vi "FlushPort.vi"(0 "reference":refnum<class "VdRs232.lvclass">, 5 "error in (no error)":errorcluster) -> (14 "duplicate reference":refnum<class "VdRs232.lvclass">, 16 "stringRead":string, 19 "error out":errorcluster)   [LabVIEW 2020, in "VdRs232.lvclass"]
doc: "Reads data from the com-port"
uses:
  VdRs232.lvclass
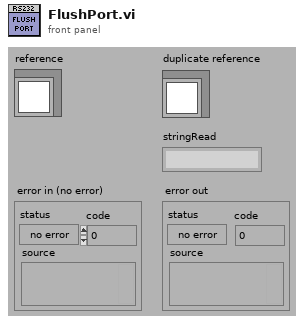
[diagram p1: front panel]
types:
  T1 = typedef "VdRs232.lvclass/ObjectAttributes.ctl" = cluster{"visaRef":refnum<visa-resource-name>, "portSetting":T2, "TimeoutTime(ms)":u32, "TerminationCharUsed":bool, "MatchPatternToIndicateCompleteResponse":string, "Creators":i32, "EndCharToSendForEveryMessage":string, "DefaultReadDataSize":u32, "SynchronousMode":bool, "Lock":T7}
  T2 = typedef "VdRs232.lvclass/ComParamsType.ctl" = cluster{"portNbr":T3, "baudRate":T4, "flowControl":T5, "parity":T6, "dataBits":u16, "stop bits (10: 1 bit)":u16}
  T3 = typedef "VdRs232.lvclass/VdRs232I_ComPortType.ctl" = enum16{"Com1", "Com2", "Com3", "Com4", "Com5", "Com6", "Com7", "Com8", "Com9", "Com10", "Com11", "Com12", "Com13", "Com14", "Com15", "Com16", "Com17", "Com18", "Com19", "Com20", "Com21", "Com22", "Com23", "Com24", "Com25", "Com26", "Com27", "Com28", "Com29", "Com30", "Com31", "Com32", "Com33", "Com34", "Com35", "Com36", "Com37", "Com38", "Com39", "Com40", "Com41", "Com42", "Com43", "Com44", "Com45", "Com46", "Com47", "Com48", "Com49", "Com50", "Com51", "Com52", "Com53", "Com54", "Com55", "Com56", "Com57", "Com58", "Com59", "Com60", "Com61", "Com62", "Com63", "Com64", "Com65", "Com66", "Com67", "Com68", "Com69", "Com70", "Com71", "Com72", "Com73", "Com74", "Com75", "Com76", "Com77", "Com78", "Com79", "Com80", "Com81", "Com82", "Com83", "Com84", "Com85", "Com86", "Com87", "Com88", "Com89", "Com90", "Com91", "Com92", "Com93", "Com94", "Com95", "Com96", "Com97", "Com98", "Com99", "Com100", "Com101", "Com102", "Com103", "Com104", "Com105", "Com106", "Com107", "Com108", "Com109", "Com110", "Com111", "Com112", "Com113", "Com114", "Com115", "Com116", "Com117", "Com118", "Com119", "Com120", "Com121", "Com122", "Com123", "Com124", "Com125", "Com126", "Com127", "Com128", "Com129", "Com130", "Com131", "Com132", "Com133", "Com134", "Com135", "Com136", "Com137", "Com138", "Com139", "Com140", "Com141", "Com142", "Com143", "Com144", "Com145", "Com146", "Com147", "Com148", "Com149", "Com150", "Com151", "Com152", "Com153", "Com154", "Com155", "Com156", "Com157", "Com158", "Com159", "Com160", "Com161", "Com162", "Com163", "Com164", "Com165", "Com166", "Com167", "Com168", "Com169", "Com170", "Com171", "Com172", "Com173", "Com174", "Com175", "Com176", "Com177", "Com178", "Com179", "Com180", "Com181", "Com182", "Com183", "Com184", "Com185", "Com186", "Com187", "Com188", "Com189", "Com190", "Com191", "Com192", "Com193", "Com194", "Com195", "Com196", "Com197", "Com198", "Com199", "Com200", "Com201", "Com202", "Com203", "Com204", "Com205", "Com206", "Com207", "Com208", "Com209", "Com210", "Com211", "Com212", "Com213", "Com214", "Com215", "Com216", "Com217", "Com218", "Com219", "Com220", "Com221", "Com222", "Com223", "Com224", "Com225", "Com226", "Com227", "Com228", "Com229", "Com230", "Com231", "Com232", "Com233", "Com234", "Com235", "Com236", "Com237", "Com238", "Com239", "Com240", "Com241", "Com242", "Com243", "Com244", "Com245", "Com246", "Com247", "Com248", "Com249", "Com250", "Com251", "Com252", "Com253", "Com254", "Com255"}
  T4 = typedef "VdRs232.lvclass/VdBaudRateType.ctl" = enum16{"1200", "2400", "9600", "14400", "19200", "28800", "38400", "57600", "115200", "230400", "460800", "691200", "921600"}
  T5 = typedef "VdRs232.lvclass/VdFlowControlType.ctl" = enum16{"None", "CTS/RTS", "XOn/XOff"}
  T6 = typedef "VdRs232.lvclass/VdParityType.ctl" = enum16{"None", "Odd", "Even"}
  T7 = typedef "Semaphore RefNum" = refnum<k1>
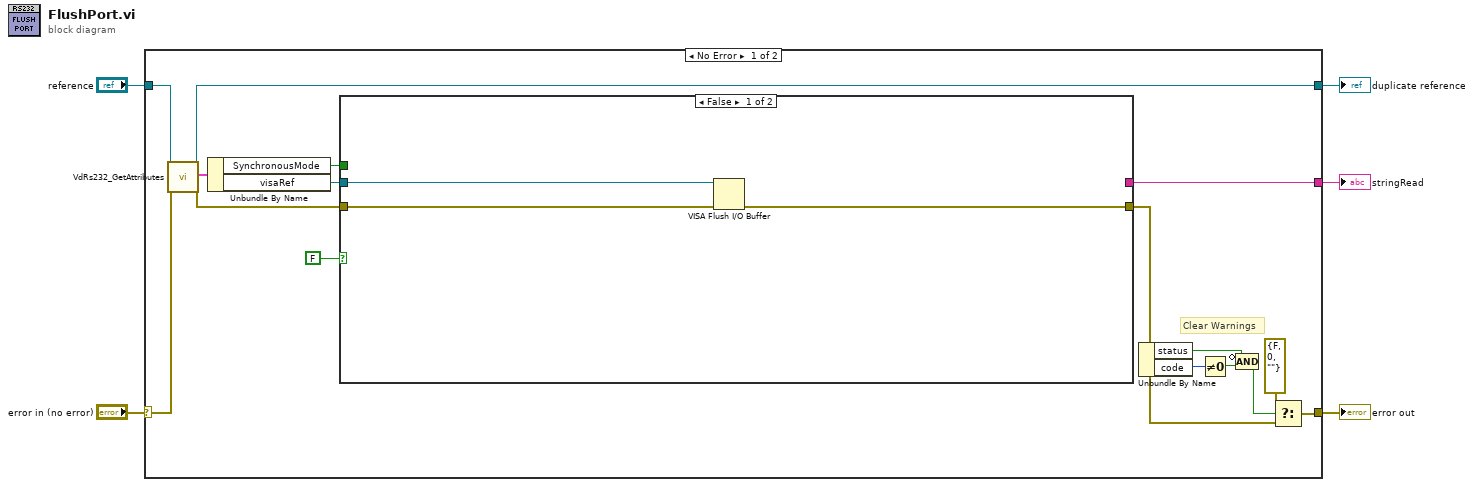
[diagram p0: block diagram]
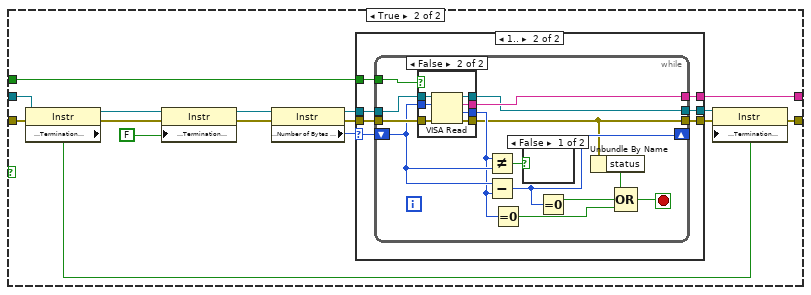
[diagram p2: hidden frame]
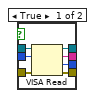
[diagram p4: hidden frame]
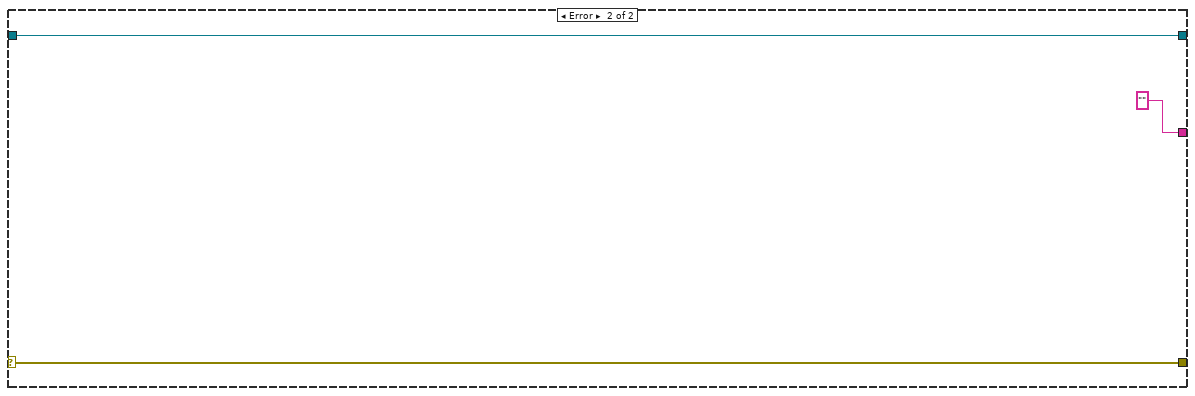
[diagram p6: hidden frame]
diagram:
  n1 = case shown="No Error" "error in (no error)" {
    selector: "error in (no error)" -> [w20 w79]
    tunnel: [w10 w79] -> w5
    tunnel: "reference" -> [w21 w80]
    tunnel: [w19 w80] -> w2
    tunnel: [w18 "" ("read buffer")] -> w1
    frame No Error {
      # "Clear Warnings"
      n2 = call "VdRs232_GetAttributes.vi"("reference in"=w21, "error in (no error)"=w20) -> ("reference out"=w19:refnum<class "VdRs232.lvclass">, "Data"=w6:T1, "error out"=w17:errorcluster)  [unwired: 1 in, 14 out]
      n3 = Unbundle By Name(w6) -> ("SynchronousMode"=w7:bool, "visaRef"=w16:refnum<visa-resource-name>)
      n4 = case shown="False" FALSE {
        tunnel: [_ w40] -> w18
        tunnel: w17 -> [w23 w39]
        tunnel: w16 -> [w24 w32]
        tunnel: [w22 w26] -> w11
        tunnel: w7 -> [_ w25]
        frame False {
          n5 = VISA Flush I/O Buffer(VISA resource name=w24, error in (no error)=w23) -> (error out=w22:errorcluster)  [unwired: 2 out]
        }
        frame True {
          n6 = property class="Instr"(reference=w32, error in=w39) -> (reference out=w30:refnum<visa-resource-name>, error out=w29:errorcluster, "Message Based Settings:Termination Character Enable"=w33:bool)
          n7 = property class="Instr"(reference=w30, error in=w29, "Message Based Settings:Termination Character Enable"=FALSE) -> (reference out=w28:refnum<visa-resource-name>, error out=w27:errorcluster)
          n8 = property class="Instr"(reference=w28, error in=w27) -> (reference out=w36:refnum<visa-resource-name>, error out=w37:errorcluster, "Serial Settings:Number of Bytes at Serial Port"=w38:u32)
          n9 = case shown="1.." w38 {
            selector: w38 -> [_ w44]
            tunnel: w36 -> [w41 w49]
            tunnel: w37 -> [w42 w48]
            tunnel: [_ w47] -> w40
            tunnel: [w42 w46] -> w34
            tunnel: [w41 w45] -> w35
            tunnel: w25 -> [_ w43]
            frame 0, Default {
            }
            frame 1.. {
              n10 = while {
                tunnel: w49 -> [w63]
                tunnel: w48 -> [w62]
                tunnel: [w61] -> w47
                tunnel: [w55] -> w46
                tunnel: [w60] -> w45
                shift-right: [w56] -> _
                shift-left: w44 -> [w58]
                tunnel: w43 -> [w50]
                stop <- w51 stop-if-true
                n11 = case shown="False" w50 {
                  tunnel: w63 -> [w70 w77]
                  tunnel: w62 -> [w69 w76]
                  tunnel: [w68 w75] -> w61
                  tunnel: [w67 w74] -> w60
                  tunnel: w58 -> [w66 w73]
                  tunnel: [w65 w72] -> w57
                  tunnel: [w64 w71] -> w55
                  frame True {
                    n12 = VISA Read(VISA resource name=w70, byte count=w66, error in (no error)=w69) -> (VISA resource name out=w67:refnum<visa-resource-name>, read buffer=w68:string, return count=w65:u32, error out=w64:errorcluster)
                  }
                  frame False {
                    n13 = VISA Read(VISA resource name=w77, byte count=w73, error in (no error)=w76) -> (VISA resource name out=w74:refnum<visa-resource-name>, read buffer=w75:string, return count=w72:u32, error out=w71:errorcluster)
                  }
                }
                n14 = Not Equal?(x=w57, y=w58) -> (x != y?=w59:bool)
                n15 = Subtract(x=w58, y=w57) -> (x-y=w56:u32)
                n16 = Equal To 0?(x=w57) -> (x = 0?=w52:bool)
                n17 = case shown="False" w59 {
                  frame False {
                  }
                  frame True {
                  }
                }
                n18 = Equal To 0?(x=w56) -> (x = 0?=w53:bool)
                n19 = Unbundle By Name(w55) -> ("status"=w54:bool)
                n20 = Compound Arithmetic op=OR(w54, w53, w52) -> (w51:bool)
              }
            }
          }
          n21 = property class="Instr"(reference=w35, error in=w34, "Message Based Settings:Termination Character Enable"=w33) -> (error out=w26:errorcluster)  [unwired: 1 out]
        }
      }
      n22 = Unbundle By Name(w11) -> ("status"=w13:bool, "code"=w15:i32)
      n23 = Not Equal To 0?(x=w15) -> (x != 0?=w14:bool)
      n24 = Compound Arithmetic op=AND(invert w13, w14) -> (w12:bool)
      n25 = Select(t=errorcluster {"status"=FALSE, "code"=0, "source"=""}, s=w12, f=w11) -> (s? t:f=w10:errorcluster)
    }
    frame Error {
    }
  }
  "error out" <- w5
  "duplicate reference" <- w2
  "stringRead" <- w1
